vi "join_arrays_replaces_join_and_fit.vi"(8 "Array to be added":dbl[][](array[numeric]), 11 "Old Array":dbl[][](array[numeric])) -> (3 "Output array":dbl[][](array[numeric]))   [LabVIEW 2021]
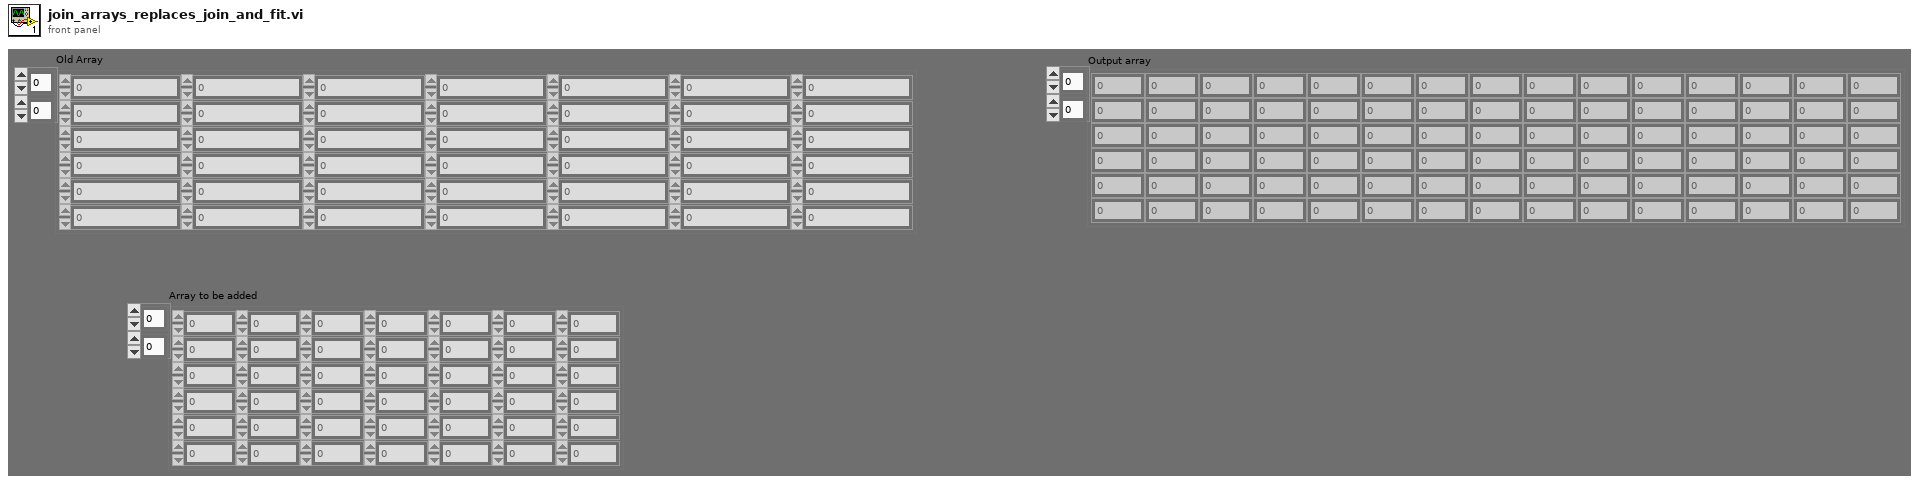
[diagram p1: front panel]
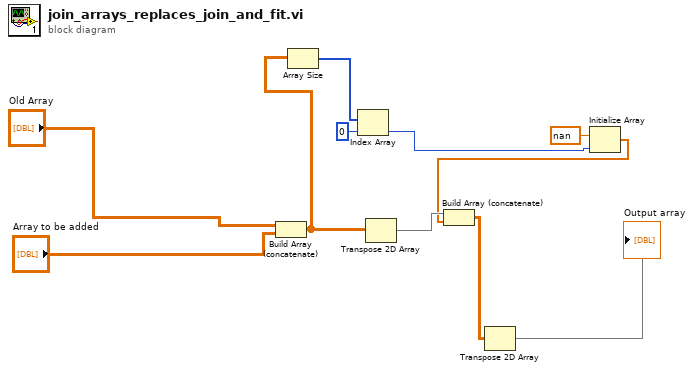
[diagram p0: block diagram]
diagram:
  n1 = Build Array (concatenate)("Old Array", "Array to be added") -> (w4:dbl[][])
  n2 = Array Size(array=w4) -> (size(s)=w11:i32[])
  n3 = Index Array(array=w11, index=0) -> (element=w8:i32)
  n4 = Transpose 2D Array(2D array=w4) -> (transposed array=w6:dbl[][])
  n5 = Initialize Array(nan ("element"), w8) -> (w5:dbl[])
  n6 = Build Array (concatenate)(w6, w5) -> (w3:dbl[][])
  n7 = Transpose 2D Array(2D array=w3) -> (transposed array=→"Output array":dbl[][])
